vi "State_Machine.vi"(8 "error in (no error)":errorcluster caption="entrée d'erreur (pas d'erreur)", 11 "Delay en entrée":refnum<class "P2056_Get_ICCID.lvclass">) -> (0 "error out":errorcluster caption="sortie d'erreur", 2 "Json_String":string, 3 "Delay en sortie":refnum<class "P2056_Get_ICCID.lvclass">)   [LabVIEW 2020, in "Library Test.lvlib" / "P2056_Get_ICCID.lvclass"]
uses:
  P2056_Get_ICCID.lvclass
  C:/Users/ngarcin/OneDrive - Altyor/Standard TB/Suite TB45/Class/Test/Test (Default)/Test (Default).lvclass
  Commun VI/TypeDef/Variable Printable.ctl
  Read CSV File/CSV_File (Default)/Class CSV_File.lvclass
  C:/Users/ngarcin/OneDrive - Altyor/Standard TB/Suite TB45/Class/Read CSV File/Class File (Default)/Class File (Default).lvclass
  JSON API/JSON Value/Set from JSON string.vi
  JSON API/JSON Value/JSON Value.lvclass
  JSON API/Variant JSON/Variant JSON.lvlib
  JSON API/Get Polymorphic/JSON GetSet.lvlib
  Commun VI/Library Commun.lvlib
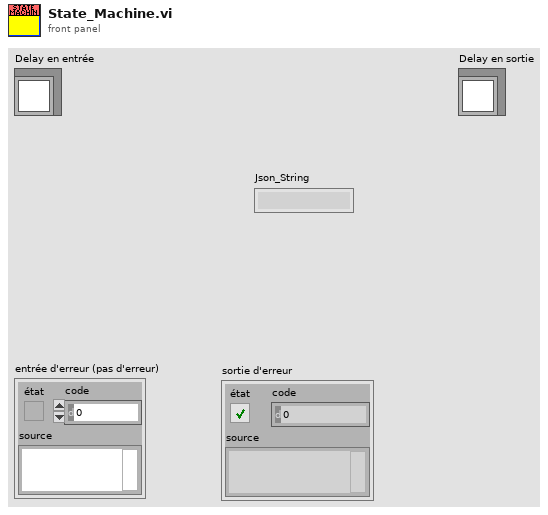
[diagram p1: front panel]
types:
  T1 = typedef "Variable Printable.ctl" = string
  T2 = enum16{"Get Variable", "Get All Variables", "Set Variable", "Delete Variable", "Delete All Variable"}
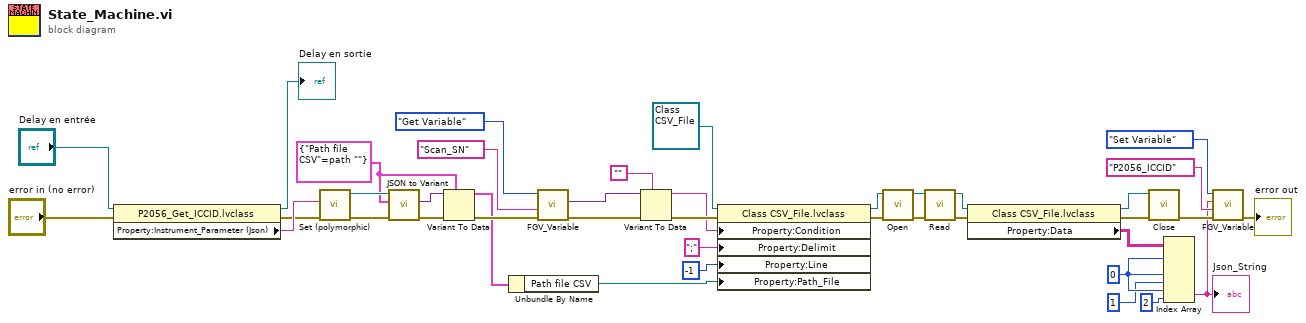
[diagram p0: block diagram]
diagram:
  w11 = 0 ("indice (ligne)")
  w32 = cluster{"Path file CSV":path} {"Path file CSV"=path ""}
  n1 = property class="P2056_Get_ICCID.lvclass"(reference="Delay en entrée", error in="error in (no error)") -> (reference out=→"Delay en sortie":refnum<class "P2056_Get_ICCID.lvclass">, error out=w33:errorcluster, "Property:Instrument_Parameter (Json)"=w35:string)
  n2 = call-poly "Set (polymorphic).vi"("error in (no error)"=w33, "JSON stream"=w35) -> ("error out"=w37:errorcluster, "JSON Value out"=w39:refnum<class "JSON Value.lvclass">)  [unwired: 7 in, 1 out]
  n3 = call "JSON to Variant.vi"("error in (no error)"=w37, "Variant (Data Type)"=w32, "JSON Value"=w39) -> ("error out"=w38:errorcluster, "Variant out"=w36:variant)  [unwired: 7 in]
  n4 = Variant To Data(error in=w38, type=w32, Variant=w36) -> (data=w19:cluster{"Path file CSV":path}, error out=w27:errorcluster)
  n5 = Unbundle By Name(w19) -> ("Path file CSV"=w13:path)
  n6 = call "FGV_Variable.vi"("error in (no error)"=w27, "Variable"=T1 "Scan_SN", "Function"=T2."Get Variable") -> ("error out"=w26:errorcluster, "Data Out"=w20:variant)  [unwired: 6 in, 1 out]
  n7 = Variant To Data(error in=w26, type="", Variant=w20) -> (data=w12:string, error out=w14:errorcluster)
  n8 = property class="Class CSV_File.lvclass"(reference=refnum<class "Class CSV_File.lvclass"> refnum ("Library File.lvlib:Class CSV_File.lvclass"), error in=w14, "Property:Condition"=w12, "Property:Delimit"=";" ("Delimit"), "Property:Line"=i16 -1 ("Line"), "Property:Path_File"=w13) -> (reference out=w16:refnum<class "Class CSV_File.lvclass">, error out=w15:errorcluster)
  n9 = call-dynamic "Open.vi"("error in (no error)"=w15, "Class CSV_File (Default) en entrée"=w16) -> ("error out"=w18:errorcluster, "Class CSV_File (Default) en sortie"=w17:refnum<class "Class CSV_File.lvclass">)  [unwired: 8 in]
  n10 = call-dynamic "Read.vi"("error in (no error)"=w18, "Class CSV_File (Default) en entrée"=w17) -> ("error out"=w24:errorcluster, "Class CSV_File (Default) en sortie"=w22:refnum<class "Class CSV_File.lvclass">)  [unwired: 8 in]
  n11 = property class="Class CSV_File.lvclass"(reference=w22, error in=w24) -> (reference out=w21:refnum<class "Class CSV_File.lvclass">, error out=w23:errorcluster, "Property:Data"=w8:string[][])
  n12 = call-dynamic "Close.vi"("error in (no error)"=w23, "Class CSV_File (Default) en entrée"=w21) -> ("error out"=w4:errorcluster)  [unwired: 8 in, 1 out]
  n13 = Index Array(array=w8, index (row) #1=w11, index (row) #2=w11, index (col) #2=1 ("indice désactivé (col)"), index (row) #3=w11, index (col) #3=2 ("indice désactivé (col)")) -> (element #3=w2:string)  [unwired: 1 in, 2 out]
  "Json_String" <- w2
  n14 = call "FGV_Variable.vi"("error in (no error)"=w4, "Variable"=T1 "P2056_ICCID", "Data In"=w2, "Function"=T2."Set Variable") -> ("error out"=→"error out":errorcluster)  [unwired: 5 in, 2 out]
